vi "SPLAT.vi"() -> ()   [LabVIEW 2014]
uses:
  Anchor/Anchor.lvclass
  Tag.lvclass
  Field Class/Field.lvclass
  Position.lvclass
panel:
  out "error out 4":errorcluster
  in  "error in (no error) 3":errorcluster
  out "ResultArray [tagID, x, y, [anchorIDarray, anchorDistancearray]":T1(array[cluster])
  out "error out 3":errorcluster
  in  "error in (no error) 2":errorcluster
  out "error out 2":errorcluster
  in  "error in (no error)":errorcluster
  out "Running":bool
  out "AnchorArray":T2(array[cluster])
  out "CombinedAnchorsArray":refnum<class "Anchor.lvclass">[](array[class])
  in  "error in":errorcluster caption="error out"
  out "error out":errorcluster
  in  "Anchors":enum32{"Page 1", "Page 4", "Page 2", "Page 3"}(tab)
  in  "Anchor 1 ID":dbl
  in  "Anchor 1 X":dbl=5.0
  in  "Anchor 1 Y":dbl=30.0
  out "Anchor 1":refnum<class "Anchor.lvclass"> caption="The result is a created anchor"
  in  "Anchor 2 ID":dbl=1.0
  in  "Anchor 2 X":dbl=60.0
  in  "Anchor 2 Y":dbl=56.0
  out "Anchor 2":refnum<class "Anchor.lvclass"> caption="The result is a created anchor"
  in  "Anchor 3 ID":dbl=2.0
  in  "Anchor 3 X":dbl=115.0
  in  "Anchor 3 Y":dbl=30.0
  out "Anchor 3":refnum<class "Anchor.lvclass"> caption="The result is a created anchor"
  out "TagsArrayInformation":cluster{"ID":dbl, "X":dbl, "Y":dbl}[](array[cluster])
  out "TagsArray":refnum<class "Tag.lvclass">[](array[class])
  in  "TraceLength":i32=10
  in  "No. players":dbl=1.0
  in  "rect":T3={"left"=10.0, "top"=55.0, "right"=110.0, "bottom"=5.0}
  in  "Input":T4={"Tag"=0.0, "X"=61.0, "Y"=30.0, "AnchorIDDistanceCluster"={"AnchorIDArray"=[], "AnchorDistanceArray"=[]}}
  in  "File path":path=path "/Macintosh HD/Users/marvineffing/Documents/SPLAT/smooth_data.txt"
  in  "Pause Button":bool
  in  "Play Button":bool
  in  "stop":bool
  in  "delay [ms]":u32=1000
  out "XY Graph":cluster{dbl[], dbl[]}[](graph)
  out "IG in":dbl[][](graph)
  out "Field":dbl[][](graph)
  # "User instructions:\nGive a file of positions for input.\nPress 'Run' button to run simulation.\nPress 'Stop' to stop simulation."
  # "TODO implement real and estimated value to be show here"
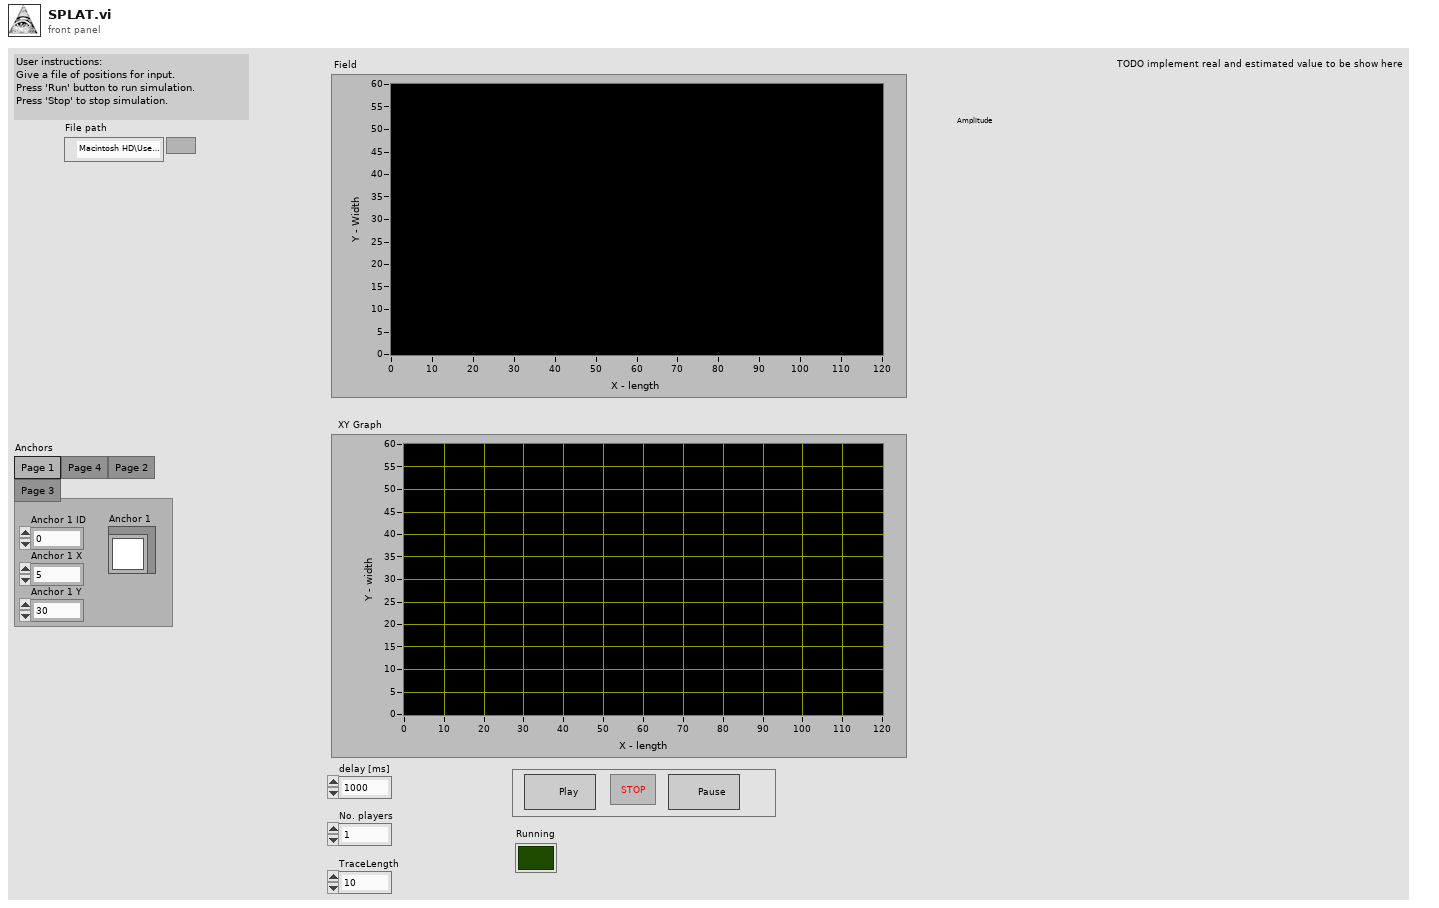
[diagram p1: front panel]
types:
  T1 = cluster{dbl, dbl, dbl, cluster{"AnchorIDArray":dbl[], "AnchorDistancesArray":dbl[]}}[]
  T2 = cluster{"AnchorID":dbl, "AnchorX":dbl, "AnchorY":dbl}[]
  T3 = cluster{"left":dbl, "top":dbl, "right":dbl, "bottom":dbl}
  T4 = cluster{"Tag":dbl, "X":dbl, "Y":dbl, "AnchorIDDistanceCluster":cluster{"AnchorIDArray":dbl[], "AnchorDistanceArray":dbl[]}}
  T5 = cluster{"TagID":dbl, "X":dbl, "Y":dbl, "AnchorIDDistanceArray":cluster{"AnchorIDArray":dbl[], "AnchorDistancesArray":dbl[]}}[]
  T6 = cluster{"Tag":dbl, "X":dbl, "Y":dbl, "Batch array":string[]}[]
  T7 = cluster{"tagID":dbl, "X":dbl, "Y":dbl, "anchorIDDistanceCluster":cluster{"anchorIDArray":dbl[], "anchorDistanceArray":dbl[]}}
  T8 = cluster{"Tag":dbl, "X":dbl, "Y":dbl, "Batch array":string[]}
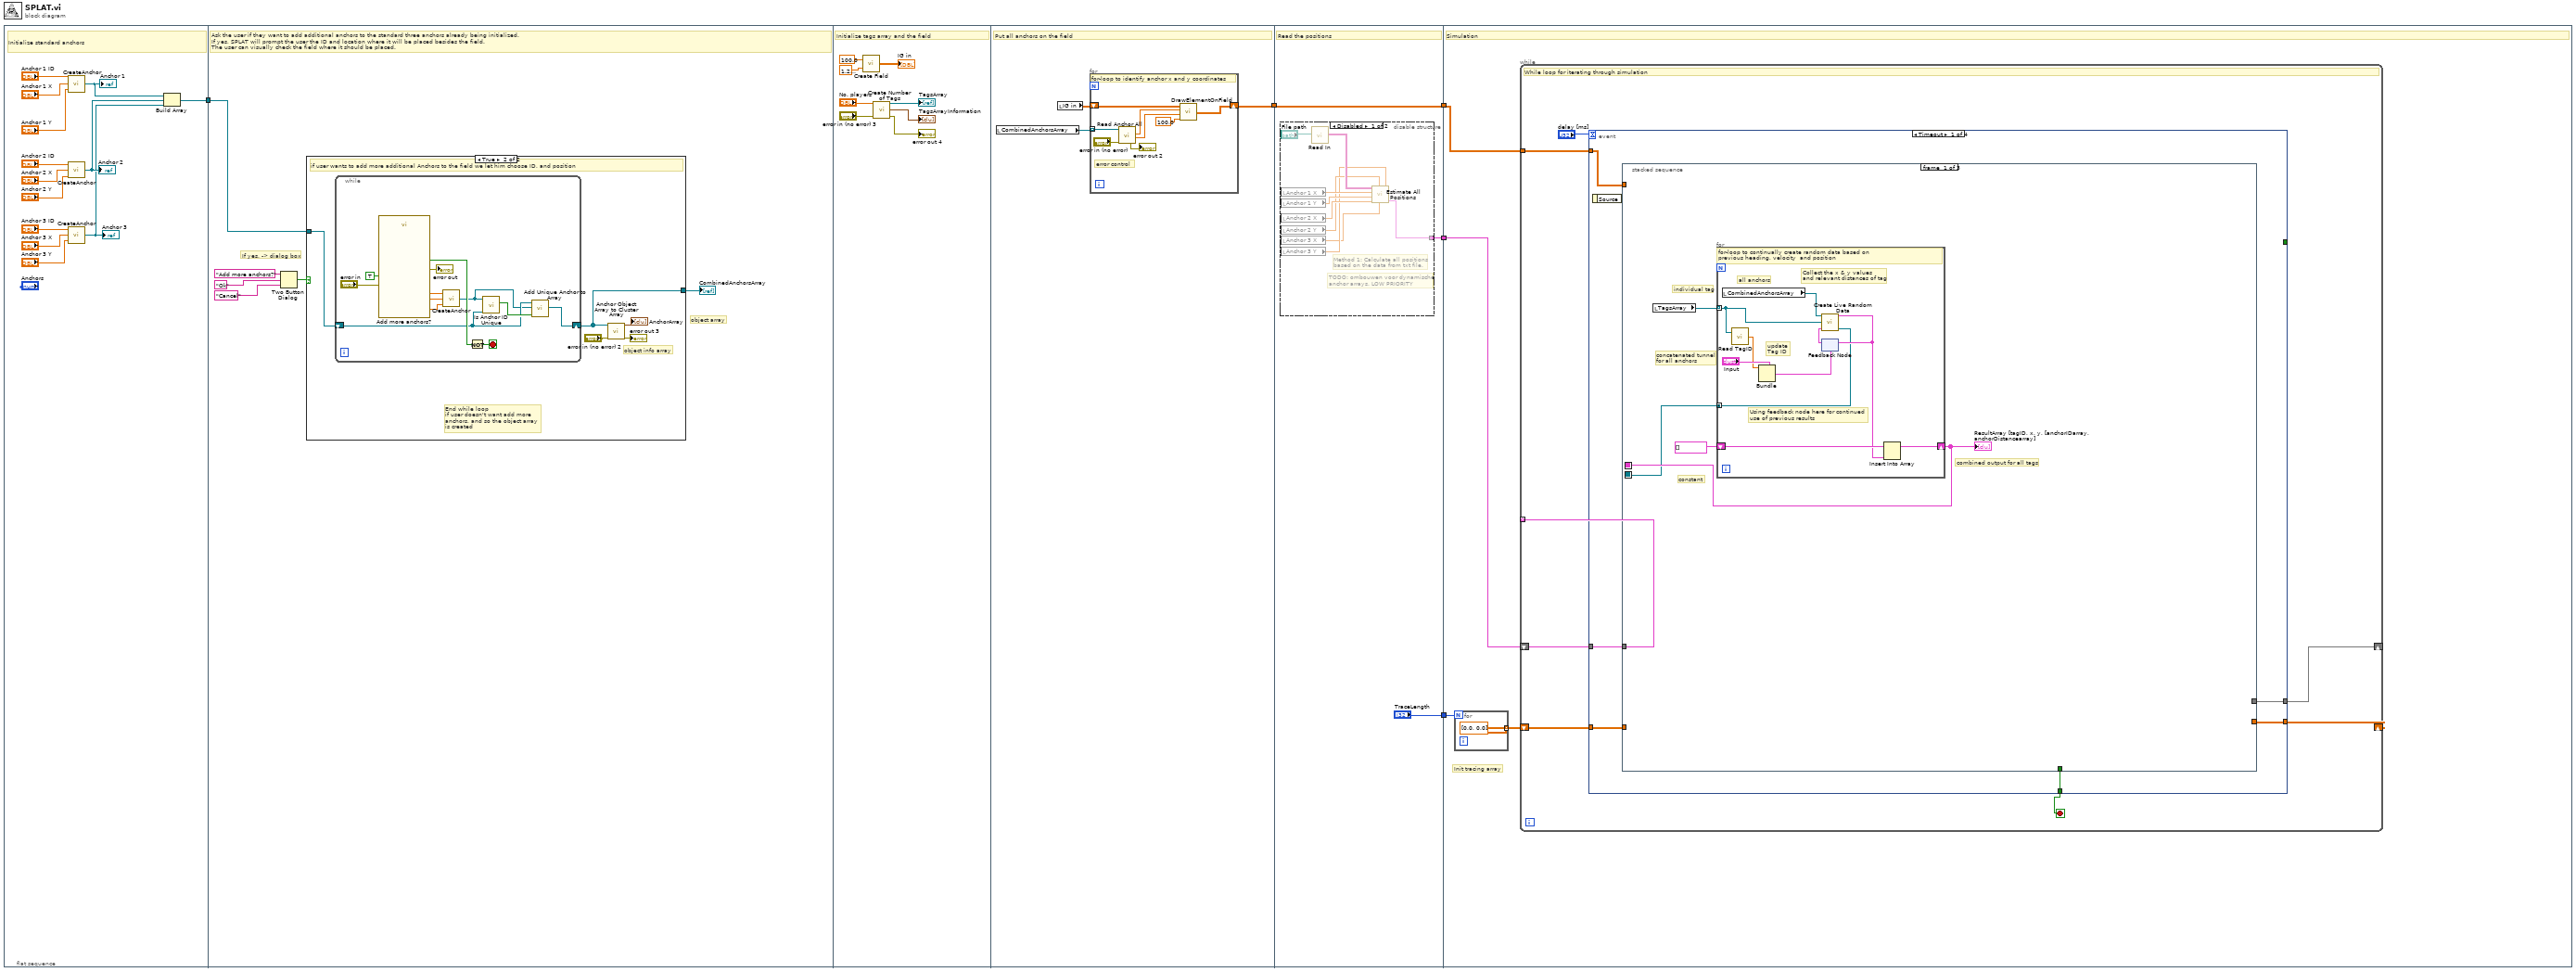
[diagram p0: block diagram]
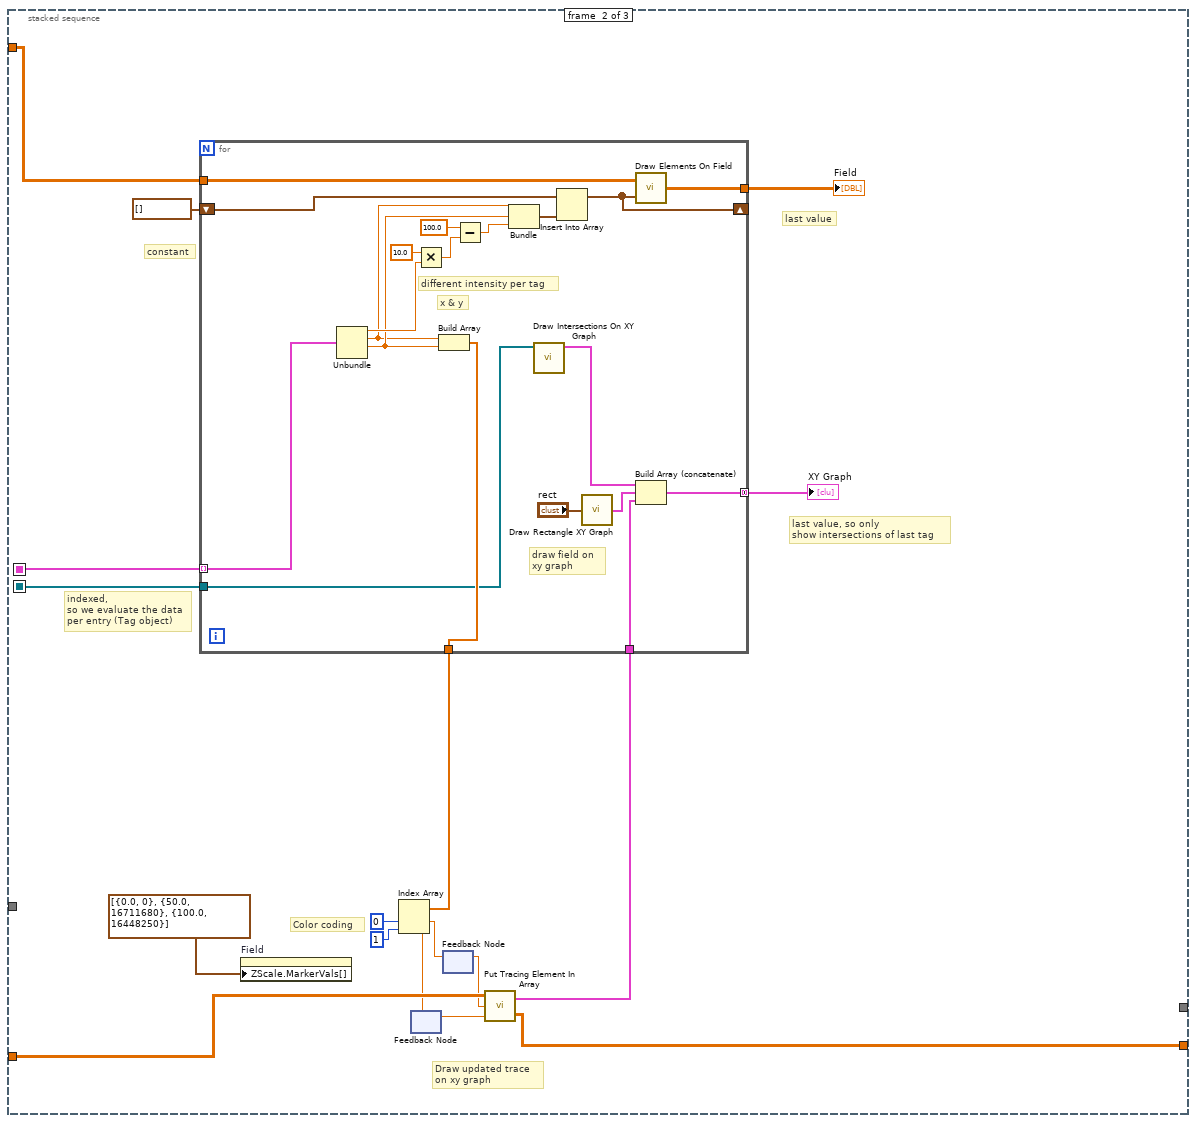
[diagram p4: hidden frame]
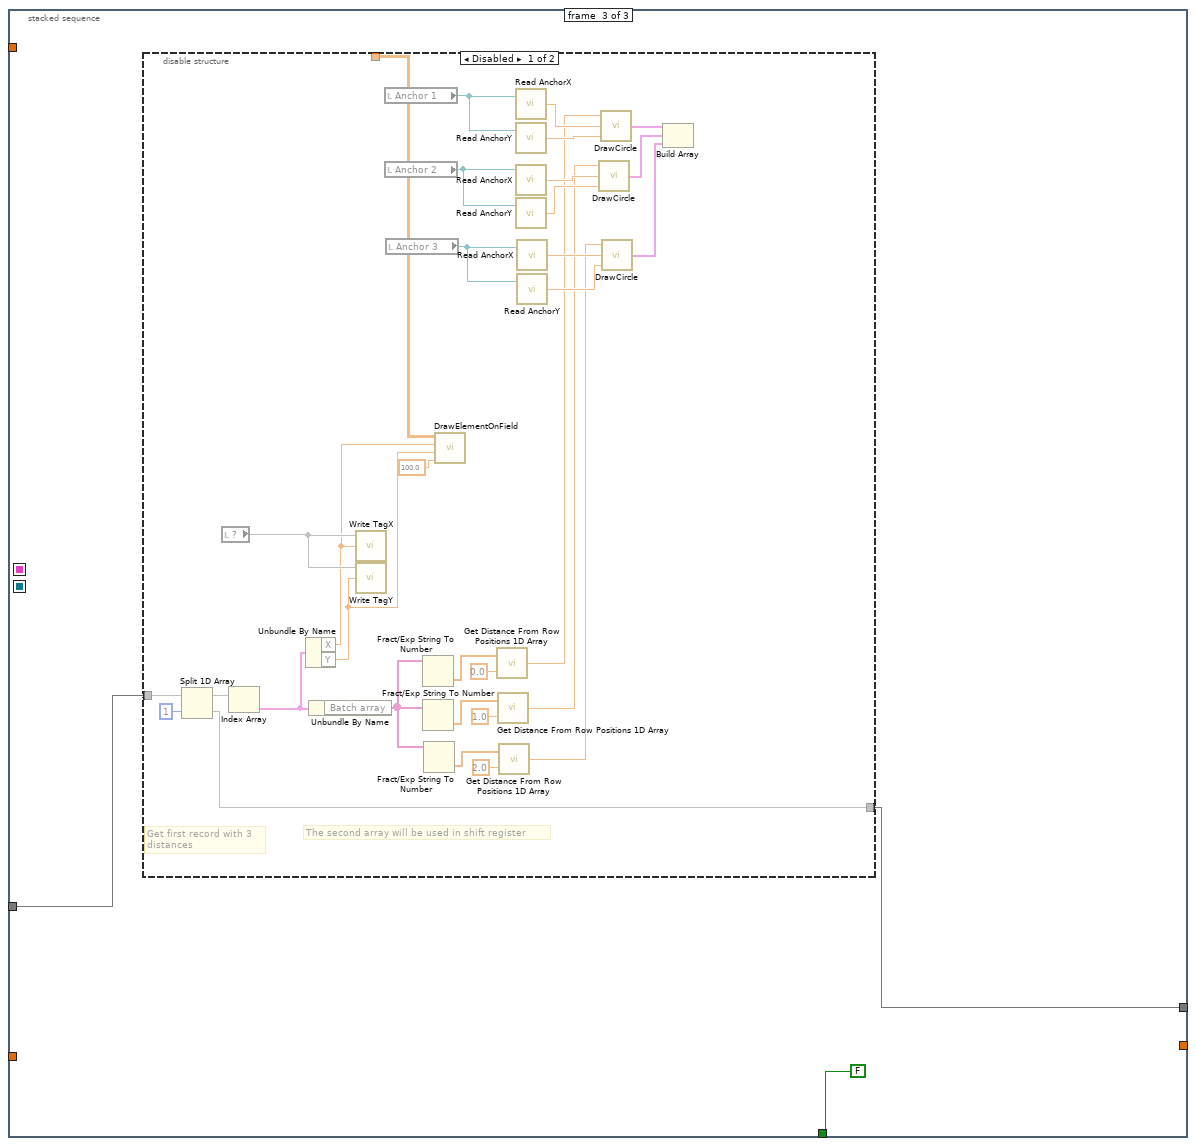
[diagram p5: hidden frame]
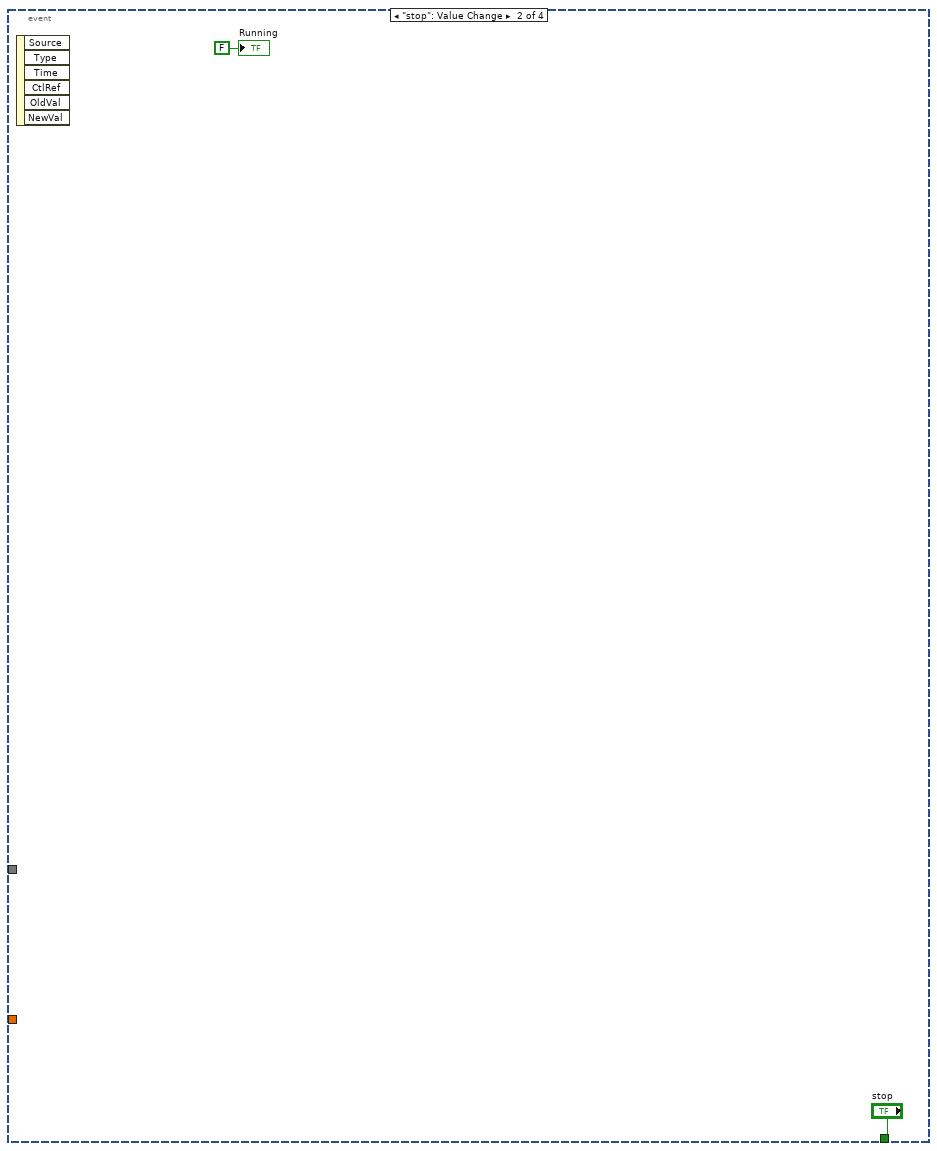
[diagram p7: hidden frame]
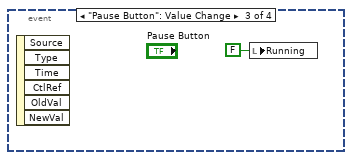
[diagram p8: hidden frame]
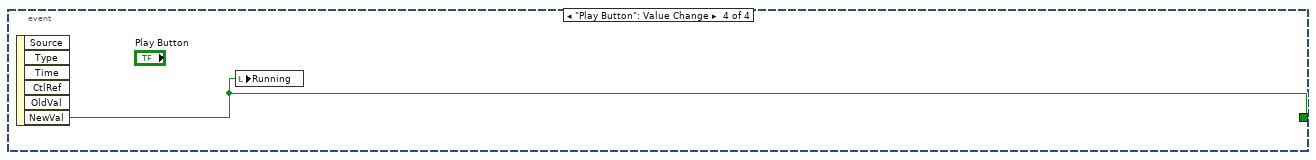
[diagram p9: hidden frame]
diagram:
  n1 = flat-sequence {
    tunnel: [w6] -> w1
    tunnel: w1 -> [w20]
    tunnel: [w52] -> w5
    tunnel: w5 -> [w64]
    tunnel: [w64] -> w4
    tunnel: [w63] -> w3
    tunnel: ["TraceLength"] -> w2
    tunnel: w4 -> [w77]
    tunnel: w3 -> [w76]
    tunnel: w2 -> [w74]
    frame #0 {
      # "Initialize standard anchors"
      n2 = call "CreateAnchor.vi"("Anchor Y"="Anchor 1 Y", "Anchor X"="Anchor 1 X", "Anchor ID"="Anchor 1 ID") -> ("Anchor Out"=w9:refnum<class "Anchor.lvclass">)
      "Anchor 1" <- w9
      n3 = call "CreateAnchor.vi"("Anchor Y"="Anchor 2 Y", "Anchor X"="Anchor 2 X", "Anchor ID"="Anchor 2 ID") -> ("Anchor Out"=w8:refnum<class "Anchor.lvclass">)
      "Anchor 2" <- w8
      n4 = call "CreateAnchor.vi"("Anchor Y"="Anchor 3 Y", "Anchor X"="Anchor 3 X", "Anchor ID"="Anchor 3 ID") -> ("Anchor Out"=w7:refnum<class "Anchor.lvclass">)
      "Anchor 3" <- w7
      n5 = Build Array(w9, w8, w7) -> (w6:refnum<class "Anchor.lvclass">[])
    }
    frame #1 {
      # "object array"
      # "If yes, -> dialog box"
      # "Ask the user if they want to add additional anchors to the standard three anchors already being initialized.\nIf yes, SPLAT will prompt the user the ID and location where it will be placed besides the field.\nThe user can visually check the field where it should be placed."
      n6 = Two Button Dialog(message="Add more anchors?", 1:"Cancel" ("F button name (\"Cancel\")"), 2:"Ok" ("T button name (\"OK\")")) -> (T button?=w21:bool)
      n7 = case shown="True" w21 {
        tunnel: w20 -> [w25 w27]
        tunnel: [w25 w26] -> w19
        frame False {
          # "do nothing\nand enter next frame"
        }
        frame True {
          # "End while loop\nif user doesn't want add more \nanchors, and so the object array \nis created"
          # "object info array"
          # "if user wants to add more additional Anchors to the field we let him choose ID, and position"
          n8 = while {
            shift-right: [w31] -> w26
            shift-left: w27 -> [w33]
            stop <- w35 stop-if-true
            n9 = call "Add more anchors?"("Enable"=TRUE, "error in (no error)"="error in") -> ("Anchor Y"=w37:dbl, "Anchor X"=w38:dbl, "Ancor ID"=w39:dbl, "Add more"=w36:bool, "error out"=→"error out":errorcluster)  [unwired: 13 in]
            n10 = call "CreateAnchor.vi"("Anchor Y"=w37, "Anchor X"=w38, "Anchor ID"=w39) -> ("Anchor Out"=w32:refnum<class "Anchor.lvclass">)
            n11 = Not(x=w36) -> (.not. x?=w35:bool)
            n12 = call "Is Anchor ID Unique.vi"("Input AnchorArray"=w33, "Anchor.lvclass"=w32) -> ("Is unique?"=w34:bool)  [unwired: 9 in]
            n13 = call "Add Unique Anchor to Array.vi"("Is Unique?"=w34, "Anchor.lvclass"=w32, "Input Anchor Array"=w33) -> ("Output Anchor Array"=w31:refnum<class "Anchor.lvclass">[])  [unwired: 8 in]
          }
          n14 = call "Anchor Object Array to Cluster Array.vi"("error in (no error)"="error in (no error) 2", "AnchorArray In"=w26) -> ("error out"=→"error out 3":errorcluster, "AnchorArray Out"=→"AnchorArray":T2)  [unwired: 8 in]
        }
      }
      "CombinedAnchorsArray" <- w19
    }
    frame #2 {
      # "Initialize tags array and the field"
      n15 = call "Create Field.vi"("RelGraphSize"=sgl 1.2, "LineIntensity"=100.0) -> ("Intensity Graph"=→"IG in":dbl[][])
      n16 = call "Create Number of Tags.vi"("NumberOfTags"="No. players", "error in (no error)"="error in (no error) 3") -> ("TagsArray"=→"TagsArray":refnum<class "Tag.lvclass">[], "TagsArrayInformation"=→"TagsArrayInformation":cluster{"ID":dbl, "X":dbl, "Y":dbl}[], "error out"=→"error out 4":errorcluster)  [unwired: 11 in]
    }
    frame #3 {
      # "Put all anchors on the field"
      n17 = local read "CombinedAnchorsArray"() -> (w51:refnum<class "Anchor.lvclass">[])
      n18 = local read "IG in"() -> (w53:dbl[][])
      n19 = for {
        tunnel: w51 -> [w55] mode=indexing
        shift-right: [w59] -> w52
        shift-left: w53 -> [w54]
        # "error control"
        # "for-loop to identify anchor x and y coordinates"
        n20 = call "Read Anchor All.vi"("error in (no error)"="error in (no error)", "Anchor in"=w55) -> ("AnchorY"=w57:dbl, "AnchorX"=w56:dbl, "error out"=→"error out 2":errorcluster)  [unwired: 4 in, 3 out]
        n21 = call "DrawElementOnField.vi"("Intensity"=100.0, "PosY"=w57, "PosX"=w56, "Field in"=w54) -> ("Field out"=w59:dbl[][])
      }
    }
    frame #4 {
      # "Read the positions"
      n22 = disable-structure shown="Disabled" {
        disable-tunnel: [w65 _] -> w63
        frame Disabled {
          # "TODO: ombouwen voor dynamische\nanchor arrays. LOW PRIORITY"
          # "Method 1: Calculate all positions\nbased on the data from txt file."
          n23 = local read "Anchor 1 X"() -> (w71:dbl)
          n24 = local read "Anchor 1 Y"() -> (w70:dbl)
          n25 = local read "Anchor 2 X"() -> (w69:dbl)
          n26 = local read "Anchor 2 Y"() -> (w68:dbl)
          n27 = local read "Anchor 3 X"() -> (w66:dbl)
          n28 = local read "Anchor 3 Y"() -> (w67:dbl)
          n29 = call "Read In.vi"("File path"="File path") -> ("DataOut [tagID, anchorID, distance, time]"=w72:string[][])
          n30 = call "Estimate All Positions.vi"("Data In [tag_id, anchor_id, distance, time]"=w72, "Anchor 2 Y"=w68, "Anchor 1 X"=w71, "Anchor 1 Y"=w70, "Anchor 3 X"=w66, "Anchor 2 X"=w69, "Anchor 3 Y"=w67) -> ("PositionsArray [tag, x,  y, distances]"=w65:T6)  [unwired: 1 out]
        }
        frame Enabled {
        }
      }
    }
    frame #5 {
      # "Init tracing array"
      # "Simulation"
      n31 = for {
        N: w74 -> [_]
        tunnel: [dbl[] [0.0, 0.0]] -> w75 mode=indexing
      }
      n32 = while {
        tunnel: w77 -> [w83]
        shift-right: [w81] -> _
        shift-left: w76 -> [w82]
        tunnel: w76 -> [_] mode=indexing
        shift-right: [w79] -> _
        shift-left: w75 -> [w80]
        stop <- w84 stop-if-true
        # "While loop for iterating through simulation"
        n33 = event shown="[0] Timeout" {
          selector: _ -> [_ _ _ _]
          dyn-events: _ -> [_ _ _ _]
          timeout: "delay [ms]" -> [_ _ _ _]
          tunnel: [w86 "stop" _ _] -> w84
          tunnel: w83 -> [w91 _ _ _]
          tunnel: w82 -> [w89 _ _ _]
          tunnel: [w88 _ _ _] -> w81
          tunnel: w80 -> [w90 _ _ _]
          tunnel: [w87 _ _ _] -> w79
          tunnel: [_ _ _ w183] -> _
          event Timeout {
            n34 = event-data() -> ()  [unwired: 1 in, 1 out]
            n35 = stacked-sequence {
              seq-local: [w93 _ _] -> [_ w121 _]
              seq-local: [w92 _ _] -> [_ w106 _]
              tunnel: [_ _ FALSE ("stop")] -> w86
              tunnel: w89 -> [_ _ w144]
              tunnel: [_ _ w143] -> w88
              tunnel: w90 -> [_ w119 _]
              tunnel: w91 -> [_ w115 _]
              tunnel: [_ w118 _] -> w87
              frame #0 {
                # "individual tag"
                # "concatenated tunnel\nfor all anchors"
                # "combined output for all tags"
                # "constant"
                n36 = local read "TagsArray"() -> (w95:refnum<class "Tag.lvclass">[])
                n37 = for {
                  tunnel: w95 -> [w100] mode=indexing
                  shift-right: [w105] -> w93
                  shift-left: T5 [] ("OutputArray") -> [w104]
                  tunnel: [w101] -> w92 mode=concatenating
                  # "update \nTag ID"
                  # "all anchors"
                  # "Collect the x & y values \nand relevant distances of tag"
                  # "Using feedback node here for continued \nuse of previous results"
                  # "for-loop to continually create random data based on \nprevious heading, velocity  and position"
                  n38 = local read "CombinedAnchorsArray"() -> (w96:refnum<class "Anchor.lvclass">[])
                  n39 = call-dynamic "Read TagID.vi"("Tag in"=w100) -> ("TagID"=w98:dbl)  [unwired: 1 in, 2 out]
                  n40 = Bundle(cluster="Input", "Tag"=w98) -> (w97:T4)  [unwired: 3 in]
                  n41 = feedback #1(w97) -> (w103:T4)
                  n42 = call "Create Live Random Data.vi"("Input AnchorArray"=w96, "Tag.lvclass"=w100, "Input"=w103) -> ("PositionOut"=w102:T7, "Output AnchorArray"=w101:refnum<class "Anchor.lvclass">[])  [unwired: 11 in]
                  n43 = feedback-in #1(w102) -> ()
                  n44 = Insert Into Array(array=w104, new element=w102) -> (w105:T5)  [unwired: 1 in]
                }
                "ResultArray [tagID, x, y, [anchorIDarray, anchorDistancearray]" <- w93
              }
              frame #1 {
                # "indexed,\nso we evaluate the data\nper entry (Tag object)"
                # "constant"
                # "last value"
                # "last value, so only\nshow intersections of last tag"
                # "Draw updated trace \non xy graph"
                # "Color coding"
                n45 = property on="Field" class="IntGraph (strict)"("ZScale.MarkerVals[]"=cluster{dbl, u32}[] [{0.0, 0}, {50.0, 16711680}, {100.0, 16448250}] ("Z Scale.Marker Values[]")) -> ()  [unwired: 2 in, 2 out]
                n46 = feedback #2() -> (w107:dbl)  [unwired: 1 in]
                n47 = feedback #3() -> (w109:dbl)  [unwired: 1 in]
                n48 = call "Put Tracing Element In Array.vi"("Y"=w107, "X"=w109, "InputTraceArray"=w119) -> ("OutputTraceArray"=w118:dbl[][], "OutputXYElement"=w116:cluster{"X":dbl[], "Y":dbl[]})
                n49 = for {
                  tunnel: w121 -> [w142] mode=indexing
                  tunnel: w115 -> [w131]
                  tunnel: [w138] -> w113
                  tunnel: [w125] -> w120 mode=concatenating
                  tunnel: [w129] -> w117
                  tunnel: w116 -> [w124]
                  shift-right: [w130] -> _
                  shift-left: cluster{"X":dbl, "Y":dbl, "Intensity":dbl}[] [] ("CoordinatesConstant") -> [w132]
                  tunnel: w106 -> [w123]
                  # "draw field on \nxy graph"
                  # "x & y"
                  # "different intensity per tag"
                  n50 = Unbundle(w142) -> ("TagID"=w140:dbl, "X"=w134:dbl, "Y"=w135:dbl)  [unwired: 1 out]
                  n51 = Multiply(x=10.0, y=w140) -> (x*y=w139:dbl)
                  n52 = Build Array(w134, w135) -> (w138:dbl[])
                  n53 = Subtract(x=100.0, y=w139) -> (x-y=w136:dbl)
                  n54 = Bundle("X"=w134, "Y"=w135, w136) -> (w133:cluster{"X":dbl, "Y":dbl, dbl})  [unwired: 1 in]
                  n55 = call "Draw Intersections On XY Graph.vi"("CombinedAnchorArray In"=w123) -> ("XY Graph Out"=w127:cluster{"x":dbl[], "y":dbl[]}[])  [unwired: 10 in]
                  n56 = Insert Into Array(array=w132, new element=w133) -> (w130:cluster{"X":dbl, "Y":dbl, "Intensity":dbl}[])  [unwired: 1 in]
                  n57 = call "Draw Rectangle XY Graph.vi"("rect"="rect") -> ("XY Graph Out"=w126:cluster{dbl[], dbl[]})
                  n58 = call "Draw Elements On Field.vi"("CoordinatesArray [x, y, intensity]"=w130, "Field In"=w131) -> ("Field Out"=w129:dbl[][])
                  n59 = Build Array (concatenate)(w127, w126, w124) -> (w125:cluster{"X":dbl[], "Y":dbl[]}[])
                }
                "XY Graph" <- w120
                "Field" <- w117
                n60 = Index Array(array=w113, index #1=0 ("index"), index #2=1 ("index")) -> (element #1=w110:dbl, element #2=w108:dbl)
                n61 = feedback-in #2(w108) -> ()
                n62 = feedback-in #3(w110) -> ()
              }
              frame #2 {
                n63 = disable-structure shown="Disabled" {
                  disable-tunnel: w144 -> [w166 _]
                  disable-tunnel: [w165 _] -> w143
                  disable-tunnel: _ -> [w150 _]
                  frame Disabled {
                    # "Get first record with 3\ndistances"
                    # "The second array will be used in shift register"
                    n64 = Split 1D Array(array=w166, index=1) -> (first subarray=w163:T6, second subarray=w165:T6)
                    n65 = local read item#-1() -> (w152)
                    n66 = Index Array(array=w163) -> (element=w151:T8)  [unwired: 1 in]
                    n67 = Unbundle By Name(w151) -> ("X"=w148:dbl, "Y"=w147:dbl)
                    n68 = Unbundle By Name(w151) -> ("Batch array"=w162:string[])
                    n69 = call-dynamic "Write TagX.vi"("TagX"=w148, "Tag in"=w152) -> ()  [unwired: 1 in, 2 out]
                    n70 = call-dynamic "Write TagY.vi"("TagY"=w147, "Tag in"=w152) -> ()  [unwired: 1 in, 2 out]
                    n71 = local read "Anchor 1"() -> (w178:refnum<class "Anchor.lvclass">)
                    n72 = local read "Anchor 2"() -> (w177:refnum<class "Anchor.lvclass">)
                    n73 = local read "Anchor 3"() -> (w176:refnum<class "Anchor.lvclass">)
                    n74 = Fract/Exp String To Number ("String > Number")(string=w162) -> (number=w157:dbl[])  [unwired: 3 in, 1 out]
                    n75 = Fract/Exp String To Number ("String > Number")(string=w162) -> (number=w158:dbl[])  [unwired: 3 in, 1 out]
                    n76 = Fract/Exp String To Number ("String > Number")(string=w162) -> (number=w156:dbl[])  [unwired: 3 in, 1 out]
                    n77 = call "DrawElementOnField.vi"("Intensity"=100.0, "PosY"=w147, "PosX"=w148, "Field in"=w150) -> ("Field out"=w149:dbl[][])
                    n78 = call "Get Distance From Row Positions 1D Array.vi"("Row"=0.0, "DistanceArray"=w157) -> ("Value"=w155:dbl)
                    n79 = call "Get Distance From Row Positions 1D Array.vi"("Row"=1.0, "DistanceArray"=w158) -> ("Value"=w154:dbl)
                    n80 = call "Get Distance From Row Positions 1D Array.vi"("Row"=2.0, "DistanceArray"=w156) -> ("Value"=w153:dbl)
                    n81 = call-dynamic "Read AnchorX.vi"("Anchor in"=w178) -> ("AnchorX"=w179:dbl)  [unwired: 1 in, 2 out]
                    n82 = call-dynamic "Read AnchorY.vi"("Anchor in"=w178) -> ("AnchorY"=w171:dbl)  [unwired: 1 in, 2 out]
                    n83 = call-dynamic "Read AnchorX.vi"("Anchor in"=w177) -> ("AnchorX"=w170:dbl)  [unwired: 1 in, 2 out]
                    n84 = call-dynamic "Read AnchorY.vi"("Anchor in"=w177) -> ("AnchorY"=w169:dbl)  [unwired: 1 in, 2 out]
                    n85 = call-dynamic "Read AnchorX.vi"("Anchor in"=w176) -> ("AnchorX"=w168:dbl)  [unwired: 1 in, 2 out]
                    n86 = call-dynamic "Read AnchorY.vi"("Anchor in"=w176) -> ("AnchorY"=w167:dbl)  [unwired: 1 in, 2 out]
                    n87 = call "DrawCircle.vi"("y"=w169, "x"=w170, "r"=w154) -> ("XY Graph"=w173:cluster{dbl[], dbl[]})
                    n88 = call "DrawCircle.vi"("y"=w171, "x"=w179, "r"=w155) -> ("XY Graph"=w175:cluster{dbl[], dbl[]})
                    n89 = call "DrawCircle.vi"("y"=w167, "x"=w168, "r"=w153) -> ("XY Graph"=w172:cluster{dbl[], dbl[]})
                    n90 = Build Array(w175, w173, w172) -> (w174:cluster{dbl[], dbl[]}[])
                  }
                  frame Enabled {
                  }
                }
              }
            }
          }
          event "stop": Value Change {
            n91 = event-data() -> ()  [unwired: 1 in, 6 out]
            "Running" <- FALSE ("Running")
          }
          event "Pause Button": Value Change {
            n92 = event-data() -> ()  [unwired: 1 in, 6 out]
            n93 = local write "Running"(FALSE ("Running")) -> ()
          }
          event "Play Button": Value Change {
            n94 = event-data() -> ("NewVal"=w183:bool)  [unwired: 1 in, 5 out]
            n95 = local write "Running"(w183) -> ()
          }
        }
      }
    }
  }
